vi "pr650_connect_blink.vi"() -> ()   [LabVIEW 2010]
uses:
  <vilib>/Waveform/WDTFileIO.llb/Export Waveforms To Spreadsheet File (1D).vi
panel:
  in  "Go Many":bool
  in  "How Many?":dbl
  out "Card Batt":bool
  out "Main Batt":bool
  out "Comm OK":bool
  in  "Connect":bool
  in  "Execute Custom command":bool
  out "VISA resource":refnum<visa-resource-name>
  out "Last measurement":cluster{"Y":dbl[], "Y":dbl[]}[](graph)
  out "data transfer":bool
  out "array":dbl[][](array[numeric])
  out "stopping":bool
  in  "Go 1!":bool
  in  "custom command":string
  out "read buffer":string
  out "bytes at port":u32
  out "return count":u32
  out "idle":bool=TRUE
  in  "stop":bool
  out "error out":errorcluster
  in  "PR650 COM port":refnum<visa-resource-name>
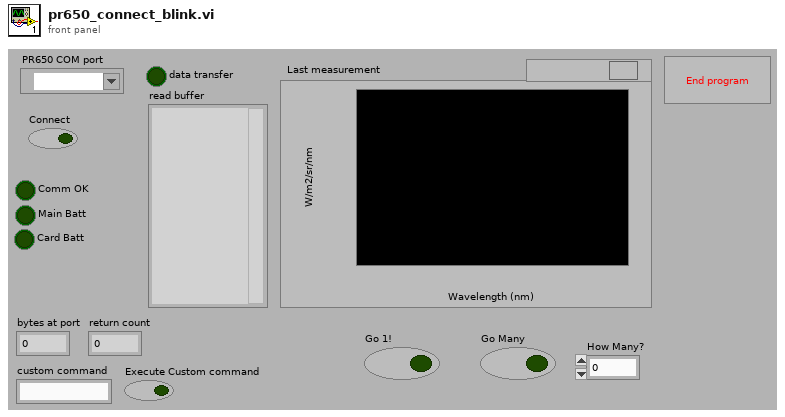
[diagram p1: front panel]
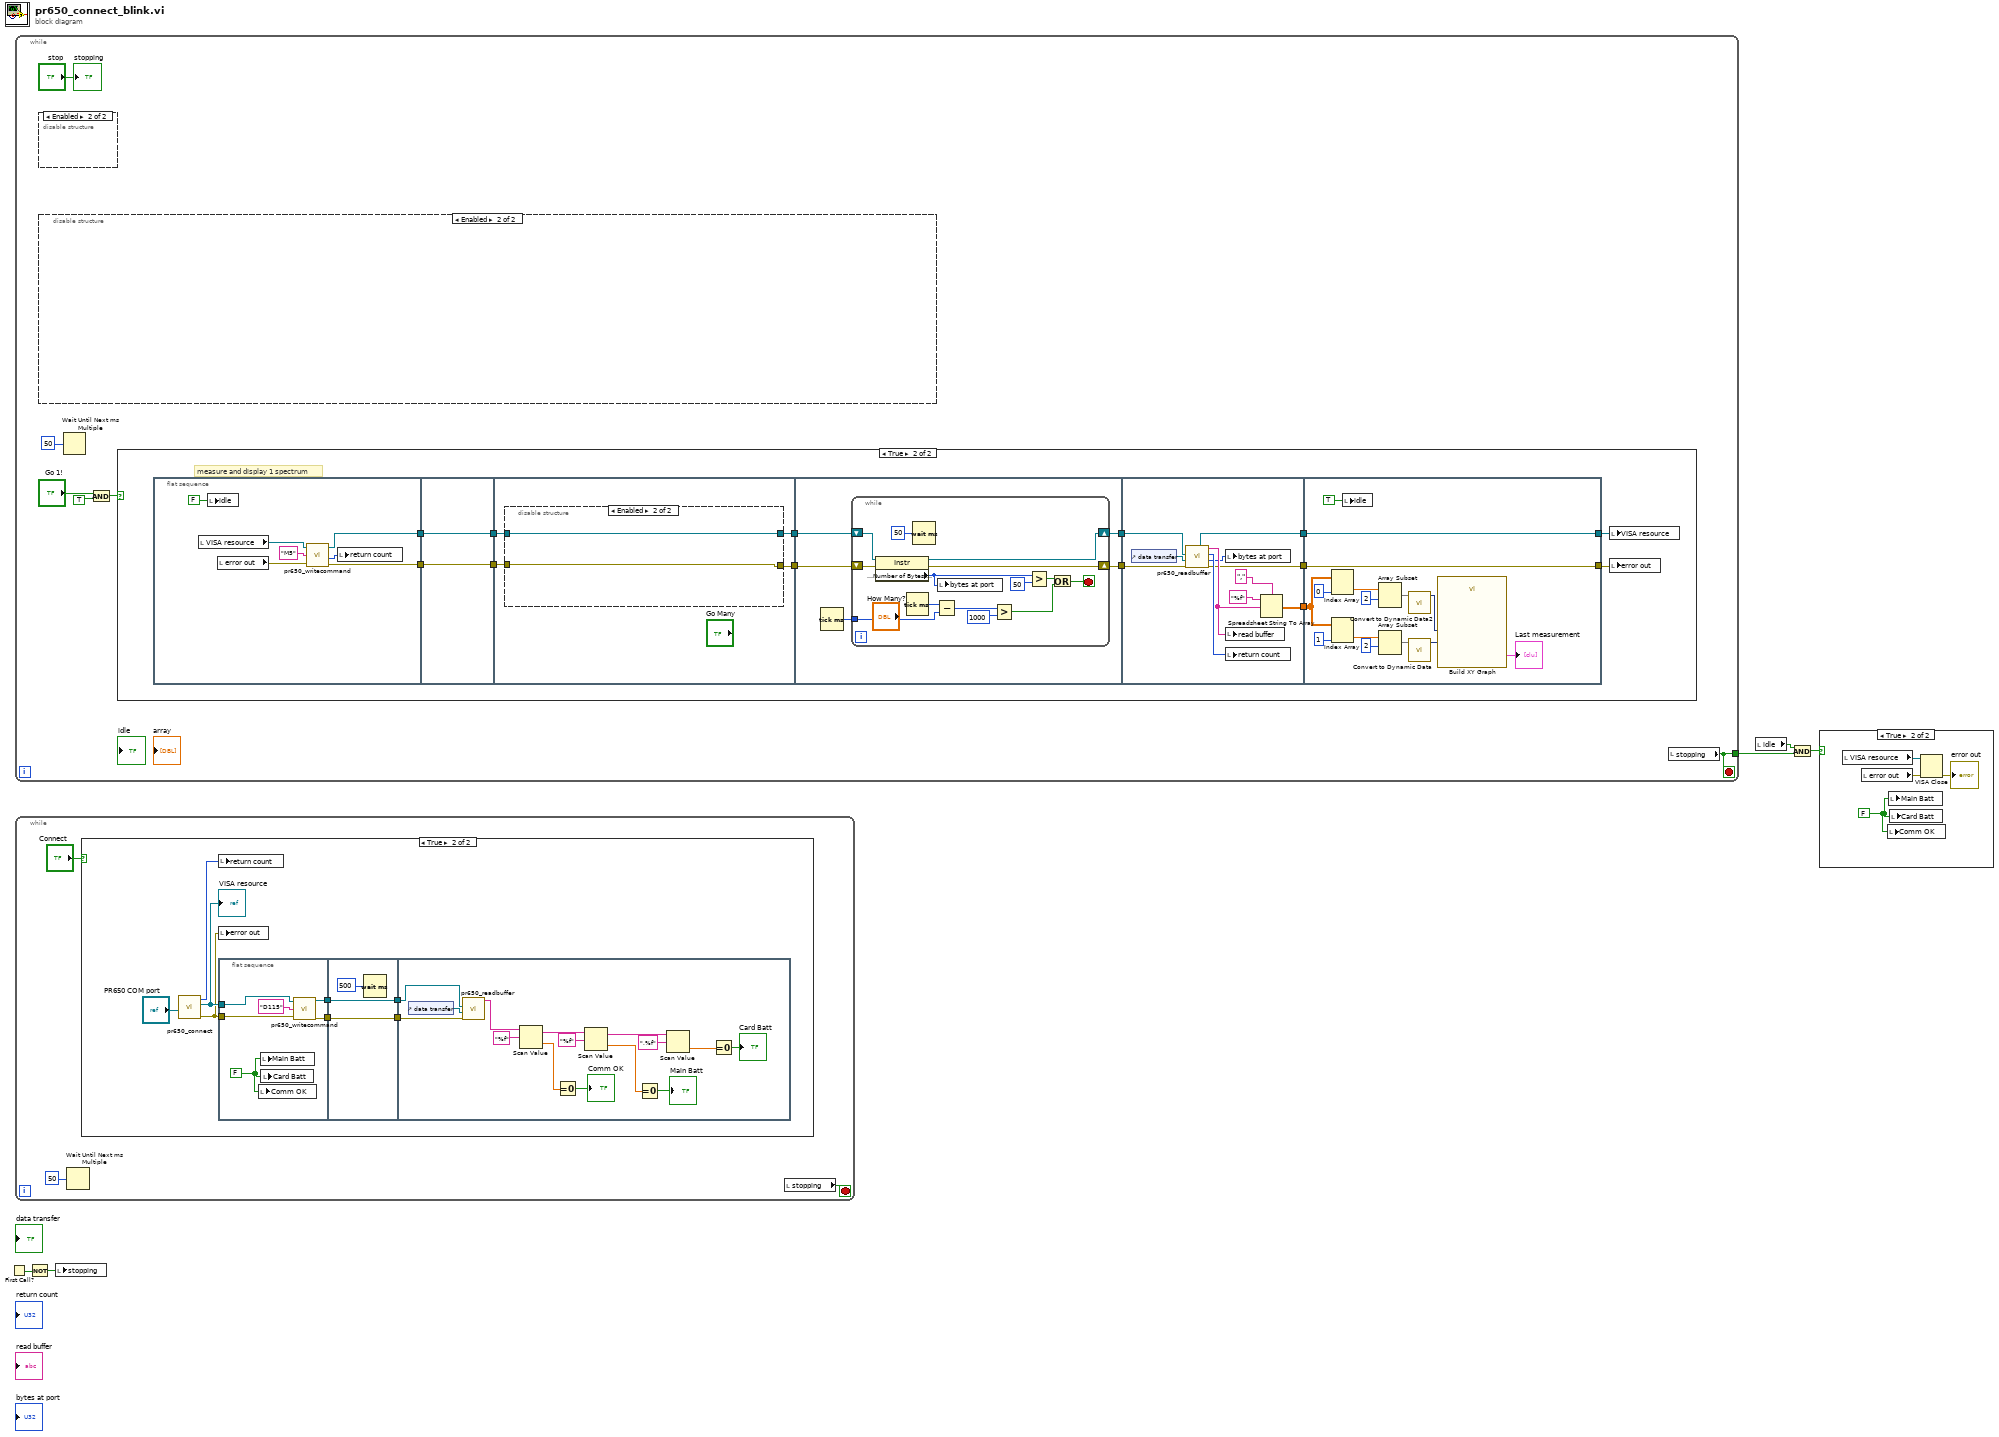
[diagram p0: block diagram]
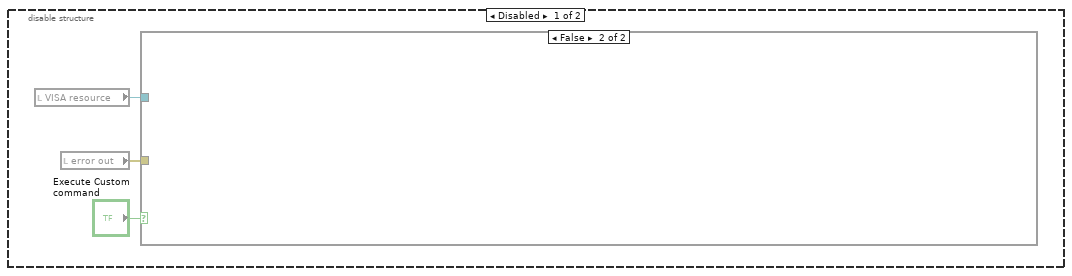
[diagram p4: hidden frame]
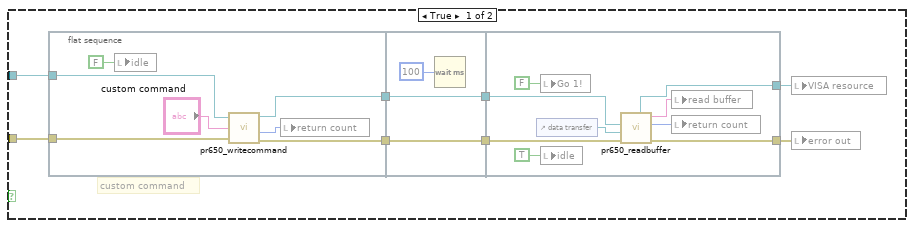
[diagram p5: hidden frame]
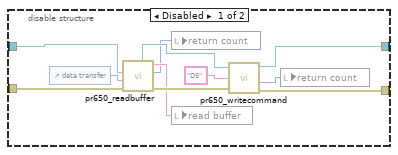
[diagram p7: hidden frame]
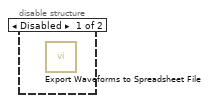
[diagram p8: hidden frame]
diagram:
  n1 = First Call?() -> (First Call?: T/F=w3:bool)
  n2 = while {
    tunnel: [w9] -> w1
    stop <- w9 stop-if-true
    n3 = disable-structure shown="Enabled" {
      frame Disabled {
        n4 = call-poly <vilib>:"Export Waveforms to Spreadsheet File.vi"() -> ()  [unwired: 10 in, 2 out]
      }
      frame Enabled {
      }
    }
    n5 = disable-structure shown="Enabled" {
      frame Disabled {
        n6 = local read "VISA resource"() -> (w14:refnum<visa-resource-name>)
        n7 = local read "error out"() -> (w13:errorcluster)
        n8 = case shown="False" "Execute Custom command" {
          tunnel: w14 -> [w16 _]
          tunnel: w13 -> [w15 _]
          frame True {
            # "custom command"
            n9 = flat-sequence {
              tunnel: [w27] -> w22
              tunnel: [w26] -> w21
              tunnel: w16 -> [w24]
              tunnel: w15 -> [w23]
              tunnel: w22 -> [w31]
              tunnel: w21 -> [w30]
              tunnel: [w31] -> w20
              tunnel: [w30] -> w19
              tunnel: [w41] -> w17
              tunnel: [w40] -> w18
              tunnel: w20 -> [w37]
              tunnel: w19 -> [w36]
              frame #0 {
                n10 = local write "idle"(FALSE ("function1")) -> ()
                n11 = call "pr650_writecommand.vi"("error in"=w23, "write buffer"="custom command", "VISA resource name in"=w24) -> ("error out"=w26:errorcluster, "return count"=w25:u32, "VISA resource name out"=w27:refnum<visa-resource-name>)  [unwired: 1 in]
                n12 = local write "return count"(w25) -> ()
              }
              frame #1 {
                n13 = Wait (ms)(milliseconds to wait=u32 100) -> ()  [unwired: 1 out]
              }
              frame #2 {
                n14 = control-ref of="data transfer"() -> (w33:refnum<vi>)
                n15 = local write "Go 1!"(FALSE ("function1")) -> ()
                n16 = local write "idle"(TRUE ("function1")) -> ()
                n17 = call "pr650_readbuffer.vi"("error in (no error)"=w36, "ref"=w33, "reference"=w37) -> ("error out"=w41:errorcluster, "return count"=w38:u32, "read buffer"=w39:string, "VISA resource name out"=w40:refnum<visa-resource-name>)  [unwired: 2 in, 1 out]
                n18 = local write "read buffer"(w39) -> ()
                n19 = local write "return count"(w38) -> ()
              }
            }
            n20 = local write "VISA resource"(w18) -> ()
            n21 = local write "error out"(w17) -> ()
          }
          frame False {
          }
        }
      }
      frame Enabled {
      }
    }
    n22 = Wait Until Next ms Multiple(millisecond multiple=u32 50) -> ()  [unwired: 1 out]
    n23 = And(x="Go 1!", y=TRUE) -> (x .and. y?=w8:bool)
    n24 = case shown="True" w8 {
      frame False {
      }
      frame True {
        # "measure and display 1 spectrum"
        n25 = flat-sequence {
          tunnel: [w60] -> w54
          tunnel: [w59] -> w53
          tunnel: w54 -> [w63]
          tunnel: w53 -> [w62]
          tunnel: [w63] -> w43
          tunnel: [w62] -> w42
          tunnel: [w66] -> w52
          tunnel: [w67] -> w47
          tunnel: w43 -> [w65]
          tunnel: w42 -> [w64]
          tunnel: w52 -> [w84]
          tunnel: [w83] -> w51
          tunnel: [w82] -> w50
          tunnel: w47 -> [w85]
          tunnel: w51 -> [w104]
          tunnel: w50 -> [w105]
          tunnel: [w103] -> w46
          tunnel: [w102] -> w45
          tunnel: [w101] -> w44
          tunnel: [w124] -> w48
          tunnel: [w125] -> w49
          tunnel: w46 -> [w125]
          tunnel: w45 -> [w124]
          tunnel: w44 -> [w112]
          frame #0 {
            n26 = local read "VISA resource"() -> (w56:refnum<visa-resource-name>)
            n27 = local write "idle"(FALSE ("function1")) -> ()
            n28 = local read "error out"() -> (w55:errorcluster)
            n29 = call "pr650_writecommand.vi"("error in"=w55, "write buffer"="M5" ("string"), "VISA resource name in"=w56) -> ("error out"=w59:errorcluster, "return count"=w58:u32, "VISA resource name out"=w60:refnum<visa-resource-name>)  [unwired: 1 in]
            n30 = local write "return count"(w58) -> ()
          }
          frame #1 {
          }
          frame #2 {
            n31 = disable-structure shown="Enabled" {
              disable-tunnel: [w76 w80] -> w67
              disable-tunnel: [w75 w79] -> w66
              disable-tunnel: w65 -> [w74 w80]
              disable-tunnel: w64 -> [w72 w79]
              frame Disabled {
                n32 = control-ref of="data transfer"() -> (w73:refnum<vi>)
                n33 = call "pr650_readbuffer.vi"("error in (no error)"=w72, "ref"=w73, "reference"=w74) -> ("error out"=w71:errorcluster, "return count"=w68:u32, "read buffer"=w69:string, "VISA resource name out"=w70:refnum<visa-resource-name>)  [unwired: 2 in, 1 out]
                n34 = local write "return count"(w68) -> ()
                n35 = local write "read buffer"(w69) -> ()
                n36 = call "pr650_writecommand.vi"("error in"=w71, "write buffer"="D5" ("string"), "VISA resource name in"=w70) -> ("error out"=w75:errorcluster, "return count"=w78:u32, "VISA resource name out"=w76:refnum<visa-resource-name>)  [unwired: 1 in]
                n37 = local write "return count"(w78) -> ()
              }
              frame Enabled {
              }
            }
          }
          frame #3 {
            n38 = Tick Count (ms)() -> (millisecond timer value=w81:u32)
            n39 = while {
              shift-right: [w99] -> w82
              shift-left: w85 -> [w97]
              shift-right: [w98] -> w83
              shift-left: w84 -> [w86]
              tunnel: w81 -> [w90]
              stop <- w92 stop-if-true
              n40 = property class="Instr"(reference=w97, error in=w86) -> (reference out=w99:refnum<visa-resource-name>, error out=w98:errorcluster, "Serial Settings:Number of Bytes at Serial Port"=w96:u32)
              n41 = Tick Count (ms)() -> (millisecond timer value=w91:u32)
              n42 = Wait (ms)(milliseconds to wait=u32 50) -> ()  [unwired: 1 out]
              n43 = Subtract(x=w91, y=w90) -> (x-y=w89:u32)
              n44 = local write "bytes at port"(w96) -> ()
              n45 = Greater?(x=w89, y=u32 1000) -> (0:w87:bool)
              n46 = Greater?(x=w96, y=u32 50) -> (0:w94:bool)
              n47 = Or(x=w94, y=w87) -> (x .or. y?=w92:bool)
            }
          }
          frame #4 {
            n48 = control-ref of="data transfer"() -> (w108:refnum<vi>)
            n49 = call "pr650_readbuffer.vi"("error in (no error)"=w104, "ref"=w108, "reference"=w105) -> ("error out"=w103:errorcluster, "bytes at port"=w100:u32, "return count"=w107:u32, "read buffer"=w106:string, "VISA resource name out"=w102:refnum<visa-resource-name>)  [unwired: 2 in]
            n50 = local write "bytes at port"(w100) -> ()
            n51 = local write "read buffer"(w106) -> ()
            n52 = local write "return count"(w107) -> ()
            n53 = Spreadsheet String To Array(delimiter (Tab)=",", format string="%f", spreadsheet string=w106) -> (array=w101:dbl[][])  [unwired: 1 in]
          }
          frame #5 {
            n54 = Index Array(array=w112, index (col)=0 ("index")) -> (element=w118:dbl[])  [unwired: 1 in]
            n55 = Index Array(array=w112, index (col)=1 ("index")) -> (element=w115:dbl[])  [unwired: 1 in]
            n56 = local write "idle"(TRUE ("function1")) -> ()
            n57 = Array Subset(array=w118, index=2) -> (w121:dbl[])  [unwired: 1 in]
            n58 = Array Subset(array=w115, index=2) -> (w120:dbl[])  [unwired: 1 in]
            n59 = call "Convert to Dynamic Data2"("Array"=w121) -> ("Dynamic Data Type"=w122:dynamicdata)  [unwired: 3 in]
            n60 = call "Convert to Dynamic Data"("Array"=w120) -> ("Dynamic Data Type"=w123:dynamicdata)  [unwired: 3 in]
            n61 = call "Build XY Graph"("Y Input"=w123, "X Input"=w122) -> ("XY Graph"=→"Last measurement":cluster{"Y":dbl[], "Y":dbl[]}[])  [unwired: 3 in, 6 out]
          }
        }
        n62 = local write "VISA resource"(w48) -> ()
        n63 = local write "error out"(w49) -> ()
      }
    }
    n64 = local read "stopping"() -> (w9:bool)
    "stopping" <- "stop"
  }
  n65 = while {
    stop <- w127 stop-if-true
    n66 = Wait Until Next ms Multiple(millisecond multiple=u32 50) -> ()  [unwired: 1 out]
    n67 = case shown="True" "Connect" {
      frame False {
      }
      frame True {
        n68 = call "pr650_connect.vi"("PR650 COM port"="PR650 COM port") -> ("error out"=w133:errorcluster, "VISA resource name out"=w134:refnum<visa-resource-name>, "return count"=w135:u32)  [unwired: 4 in]
        "VISA resource" <- w134
        n69 = local write "return count"(w135) -> ()
        n70 = local write "error out"(w133) -> ()
        n71 = flat-sequence {
          tunnel: w134 -> [w141]
          tunnel: w133 -> [w140]
          tunnel: [w139] -> w131
          tunnel: [w138] -> w130
          tunnel: [w144] -> w132
          tunnel: w131 -> [w144]
          tunnel: w130 -> [w143]
          tunnel: [w143] -> w129
          tunnel: w132 -> [w159]
          tunnel: w129 -> [w158]
          frame #0 {
            w137 = FALSE
            n72 = local write "Comm OK"(w137) -> ()
            n73 = local write "Main Batt"(w137) -> ()
            n74 = local write "Card Batt"(w137) -> ()
            n75 = call "pr650_writecommand.vi"("error in"=w140, "write buffer"="D115" ("string"), "VISA resource name in"=w141) -> ("error out"=w138:errorcluster, "VISA resource name out"=w139:refnum<visa-resource-name>)  [unwired: 1 in, 1 out]
          }
          frame #1 {
            n76 = Wait (ms)(milliseconds to wait=u32 500) -> ()  [unwired: 1 out]
          }
          frame #2 {
            n77 = control-ref of="data transfer"() -> (w160:refnum<vi>)
            n78 = call "pr650_readbuffer.vi"("error in (no error)"=w158, "ref"=w160, "reference"=w159) -> ("read buffer"=w157:string)  [unwired: 2 in, 4 out]
            n79 = Scan Value(string=w157, format string="%f") -> (output string=w154:string, value=w155:dbl)  [unwired: 1 in]
            n80 = Equal To 0?(x=w155) -> (x = 0?=→"Comm OK":bool)
            n81 = Scan Value(string=w154, format string="%f") -> (output string=w151:string, value=w149:dbl)  [unwired: 1 in]
            n82 = Equal To 0?(x=w149) -> (x = 0?=→"Main Batt":bool)
            n83 = Scan Value(string=w151, format string=",%f") -> (value=w146:dbl)  [unwired: 1 in, 1 out]
            n84 = Equal To 0?(x=w146) -> (x = 0?=→"Card Batt":bool)
          }
        }
      }
    }
    n85 = local read "stopping"() -> (w127:bool)
  }
  n86 = Not(x=w3) -> (.not. x?=w2:bool)
  n87 = local write "stopping"(w2) -> ()
  n88 = local read "idle"() -> (w5:bool)
  n89 = Compound Arithmetic op=AND(w5, w1) -> (w4:bool)
  n90 = case shown="True" w4 {
    frame False {
    }
    frame True {
      w161 = FALSE
      n91 = local read "VISA resource"() -> (w163:refnum<visa-resource-name>)
      n92 = local read "error out"() -> (w162:errorcluster)
      n93 = local write "Comm OK"(w161) -> ()
      n94 = local write "Main Batt"(w161) -> ()
      n95 = local write "Card Batt"(w161) -> ()
      n96 = VISA Close(VISA resource name=w163, error in (no error)=w162) -> (error out=→"error out":errorcluster)
    }
  }
